vi "dc2ac.vi"(2 "Efficiency [pu]":dbl format="%#_13g", 3 "Pdc":dbl format="%#_13g") -> (0 "Pac":dbl format="%#_13g")   [LabVIEW 2021]
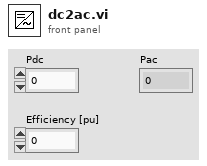
[diagram p1: front panel]
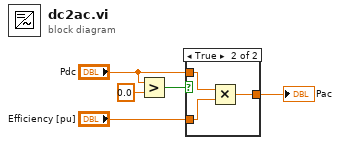
[diagram p0: block diagram]
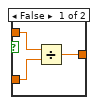
[diagram p2: hidden frame]
diagram:
  n1 = Greater?(x="Pdc", y=0.0) -> (0:w4:bool)
  n2 = case shown="True" w4 {
    tunnel: [w8 w9] -> w3
    tunnel: "Pdc" -> [w7 w11]
    tunnel: "Efficiency [pu]" -> [w6 w10]
    frame False {
      n3 = Divide(x=w7, y=w6) -> (x/y=w8:dbl)
    }
    frame True {
      n4 = Multiply(x=w11, y=w10) -> (x*y=w9:dbl)
    }
  }
  "Pac" <- w3
